vi "Write Port.vi"(0 "Simulated Device in":refnum<class "Simulated Device.lvclass">, 5 "VISA resource name":refnum<visa-resource-name>, 7 "Binary Number":T1, 9 "Port 2":dbl, 11 "error in (no error)":errorcluster) -> (4 "Simulated Device out":refnum<class "Simulated Device.lvclass">, 8 "VISA resource name 2":refnum<visa-resource-name>, 10 "Response":string, 15 "error out":errorcluster)   [LabVIEW 2020, in "Simulated Device.lvclass"]
uses:
  Simulated Device.lvclass
  Abstract/Serial Device/Serial Device.lvclass
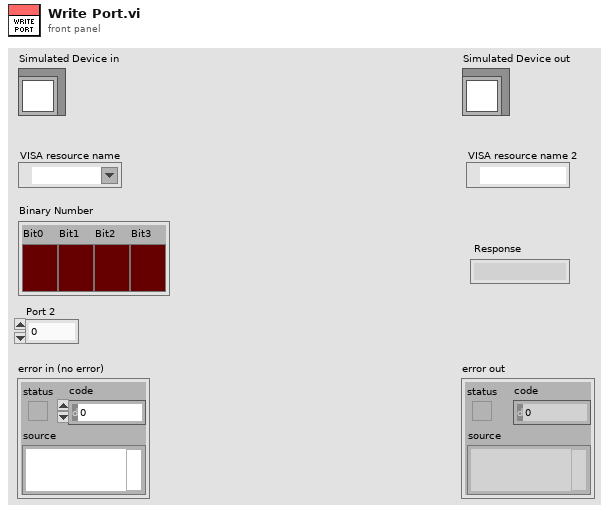
[diagram p1: front panel]
types:
  T1 = cluster{"Bit0":bool, "Bit1":bool, "Bit2":bool, "Bit3":bool}
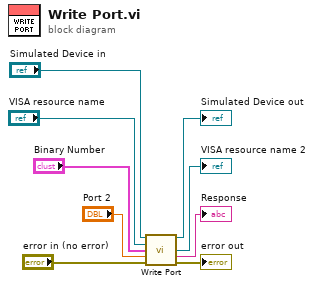
[diagram p0: block diagram]
diagram:
  n1 = call-parent "Write Port.vi"("Serial Device in"="Simulated Device in", "VISA resource name"="VISA resource name", "Binary Number"="Binary Number", "Port 2"="Port 2", "error in (no error)"="error in (no error)") -> ("Serial Device out"=→"Simulated Device out":refnum<class "Simulated Device.lvclass">, "VISA resource name 2"=→"VISA resource name 2":refnum<visa-resource-name>, "Response"=→"Response":string, "error out"=→"error out":errorcluster)  [unwired: 7 in]
